vi "Joystick 2 ArmCurlSystem.vi"(10 "Secondary Joystick Buttons":bool[](array[boolean]), 11 "Secondary Joystick Values":dbl[](array[numeric])) -> (0 "Reset Arm Encoders":bool, 1 "Arm Down":bool, 2 "Arm Up":bool, 3 "Shoulder Speed":dbl)   [LabVIEW 2018]
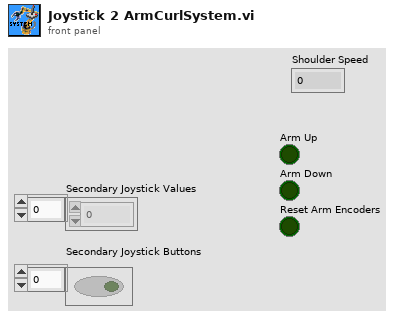
[diagram p1: front panel]
types:
  T1 = typedef "SecondaryJoystickButtons.ctl" = cluster{"Intake":bool, "Outtake":bool, "Arm Up":bool, "Arm Down":bool, "Open Grip":bool, "Close Grip":bool, "Climber Up":bool, "Climber Down":bool, "Reset Climber Encoder":bool}
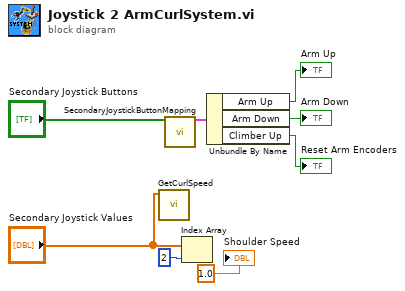
[diagram p0: block diagram]
diagram:
  n1 = call "GetCurlSpeed.vi"("SecondaryJoystickValues"="Secondary Joystick Values") -> ()  [unwired: 10 in, 1 out]
  n2 = call "SecondaryJoystickButtonMapping.vi"("Secondary joystick buttons"="Secondary Joystick Buttons") -> ("SecondaryJoystickButtons"=w7:T1)  [unwired: 13 in, 1 out]
  n3 = Index Array(array="Secondary Joystick Values", index=2) -> ()  [unwired: 1 out]
  n4 = Unbundle By Name(w7) -> ("Arm Up"=→"Arm Up":bool, "Arm Down"=→"Arm Down":bool, "Climber Up"=→"Reset Arm Encoders":bool)
  "Shoulder Speed" <- 1.0 ("Shoulder Speed")
